vi "Grafos.vi"() -> ()   [LabVIEW 2020]
uses:
  <vilib>/measure/NI_MABase.lvlib
panel:
  in  "stop":bool
  out "Waveform Chart 4":waveform(dbl)(graph)
  out "Waveform Chart 3":waveform(dbl)(graph)
  out "Waveform Chart 2":waveform(dbl)(graph)
  out "Waveform Chart":waveform(dbl)(graph)
  in  "Frecuecia":dbl(slide) scale=0.0..60.0
  in  "Amplitud":dbl(slide) scale=0.0..220.0
  # "1"
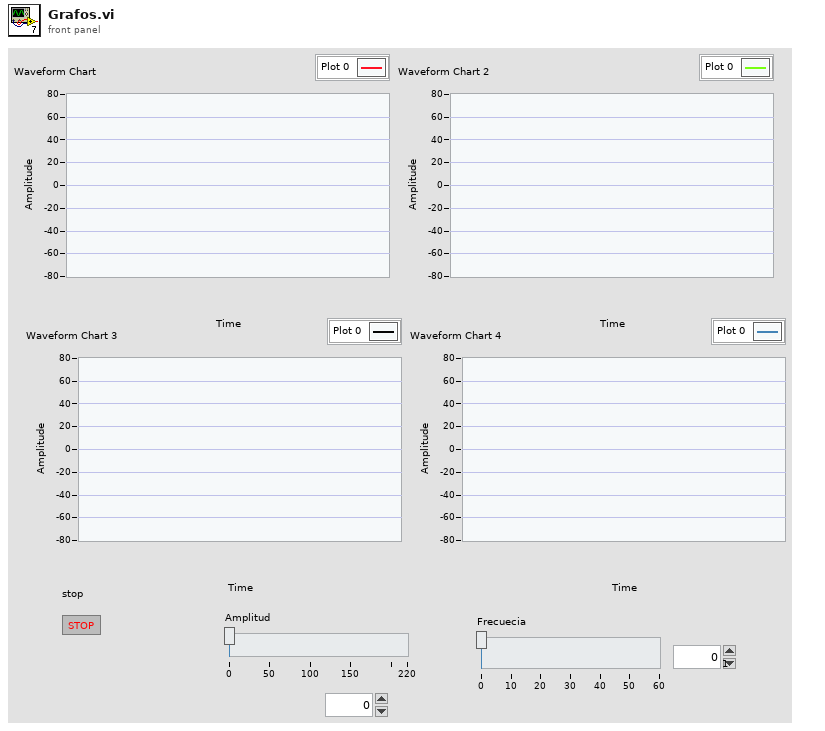
[diagram p1: front panel]
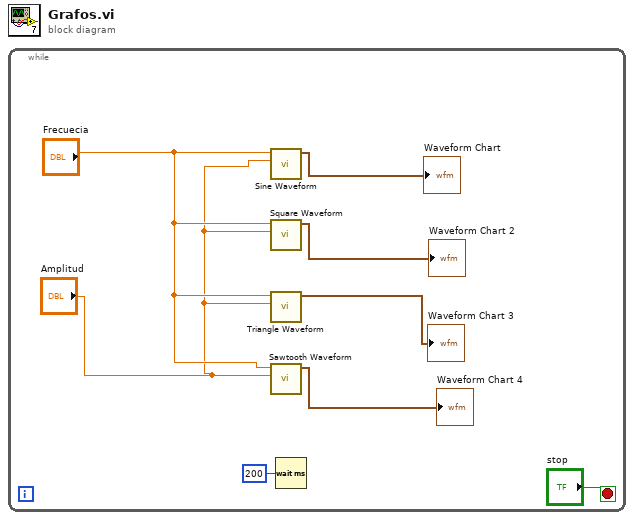
[diagram p0: block diagram]
diagram:
  n1 = while {
    stop <- "stop" stop-if-true
    n2 = call <vilib>:"Sine Waveform.vi"("amplitude"="Amplitud", "frequency"="Frecuecia") -> ("signal out"=→"Waveform Chart":waveform(dbl))  [unwired: 8 in, 1 out]
    n3 = call <vilib>:"Square Waveform.vi"("amplitude"="Amplitud", "frequency"="Frecuecia") -> ("signal out"=→"Waveform Chart 2":waveform(dbl))  [unwired: 8 in, 1 out]
    n4 = call <vilib>:"Triangle Waveform.vi"("amplitude"="Amplitud", "frequency"="Frecuecia") -> ("signal out"=→"Waveform Chart 3":waveform(dbl))  [unwired: 8 in, 1 out]
    n5 = call <vilib>:"Sawtooth Waveform.vi"("amplitude"="Amplitud", "frequency"="Frecuecia") -> ("signal out"=→"Waveform Chart 4":waveform(dbl))  [unwired: 8 in, 1 out]
    n6 = Wait (ms)(milliseconds to wait=u32 200) -> ()  [unwired: 1 out]
  }
